vi "PixieDownloadBoot.vi"(6 "Offline analysis ?":bool, 7 "PixieBootFilePaths":T1={"Communication FPGA file for REVB (.bin file in folder \"Firmware\")"=path "C:/XIA/Pixie4/Firmware/syspixie_RevB.bin", "Communication FPGA file for REVC (.bin file in folder \"Firmware\")"=path "C:/XIA/Pixie4/Firmware/syspixie_revC.bin", "Signal proceesing FPGA file (.bin file in folder \"Firmware\")"=path "C:/XIA/Pixie4/Firmware/pixie.bin", "DSP executable code file (.bin file in folder DSP\")"=path "C:/XIA/Pixie4/DSP/PXIcode.bin", "DSP parameters file (.set file in folder \"Configuration\")"=path "C:/XIA/Pixie4/Configuration/BouncerHighNoiseDec12.txt", "DSP I/O variable file (.var file in folder \"DSP\")"=path "C:/XIA/Pixie4/DSP/PXIcode.var", "DSP memory variable file (.lst file in folder \"DSP\")"=path "C:/XIA/Pixie4/DSP/PXIcode.lst"}, 8 "error in (no error)":errorcluster, 9 "Select PXI chassis type":string(combo)="4 or 8-slot chassis", 10 "Module #":u16[](array[numeric])=[2, 3] caption="PXI Slot #" min=2 max=18 step=1, 11 "Total number of Pixie-4 modules":u16=1 min=1 max=17 step=1) -> (0 "error out":errorcluster, 3 "Return value for booting":i32)   [LabVIEW 2013, in "PixieDriver.lvlib"]
uses:
  PixieDriver.lvlib
  XIA/Pixie4/Drivers/Pixie4DLL.dll
panel:
  # "0  - boot successful\n-1  - unable to scan the PXI crate slots\n-2  - unable to read communication FPGA configuration (Rev. B)\n-3  - unable to read communication FPGA configuration (Rev. C)\n-4  - unable to read signal processing FPGA configuration\n-5  - unable to read DSP executable code\n-6  - unable to read DSP parameter values\n-7  - unable to initialize DSP parameter names\n-8  - failed to boot all modules present in the system\n-9  - failed to initialize NUMBER_MODULES\n-10- failed to initialize OFFLINE_ANALYSIS\n-11- failed to initialize MAX_NUMBER_MODULES\n-12- failed to initialize SLOT_WAVE"
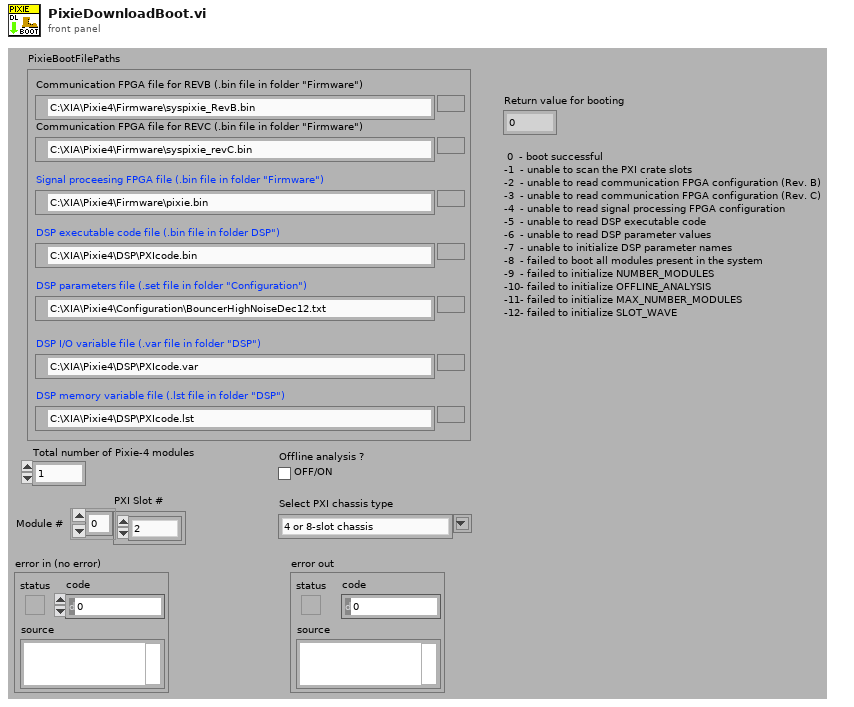
[diagram p1: front panel]
types:
  T1 = cluster{"Communication FPGA file for REVB (.bin file in folder \"Firmware\")":path, "Communication FPGA file for REVC (.bin file in folder \"Firmware\")":path, "Signal proceesing FPGA file (.bin file in folder \"Firmware\")":path, "DSP executable code file (.bin file in folder DSP\")":path, "DSP parameters file (.set file in folder \"Configuration\")":path, "DSP I/O variable file (.var file in folder \"DSP\")":path, "DSP memory variable file (.lst file in folder \"DSP\")":path}
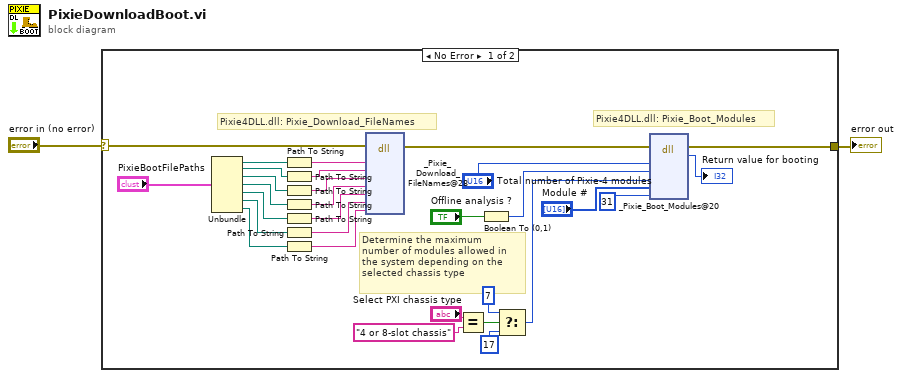
[diagram p0: block diagram]
diagram:
  n1 = case shown="No Error" "error in (no error)" {
    selector: "error in (no error)" -> [w3 w33]
    tunnel: [w4 w33] -> w2
    frame No Error {
      # "Pixie4DLL.dll: Pixie_Boot_Modules"
      # "Determine the maximum\nnumber of modules allowed in\nthe system depending on the\nselected chassis type"
      # "Pixie4DLL.dll: Pixie_Download_FileNames"
      n2 = Unbundle("PixieBootFilePaths") -> ("Communication FPGA file for REVB (.bin file in folder \"Firmware\")"=w11:path, "Communication FPGA file for REVC (.bin file in folder \"Firmware\")"=w10:path, "Signal proceesing FPGA file (.bin file in folder \"Firmware\")"=w9:path, "DSP executable code file (.bin file in folder DSP\")"=w8:path, "DSP parameters file (.set file in folder \"Configuration\")"=w7:path, "DSP I/O variable file (.var file in folder \"DSP\")"=w6:path, "DSP memory variable file (.lst file in folder \"DSP\")"=w5:path)
      n3 = Path To String(path=w11) -> (string=w26:string)
      n4 = Path To String(path=w10) -> (string=w27:string)
      n5 = Path To String(path=w9) -> (string=w28:string)
      n6 = Path To String(path=w8) -> (string=w29:string)
      n7 = Path To String(path=w7) -> (string=w30:string)
      n8 = Path To String(path=w6) -> (string=w31:string)
      n9 = Path To String(path=w5) -> (string=w32:string)
      n10 = dll-call lib="C:/XIA/Pixie4/Drivers/Pixie4DLL.dll" fn="_Pixie_Download_FileNames@28" ("Call Library Function")(error in=w3, "ComFPGAFileNameRevB"=w26, "ComFPGAFileNameRevC"=w27, "SPFPGAFileName"=w28, "DSPCodeFileName"=w29, "DSPParFileName"=w30, "DSPVarFileName"=w31, "DSPLstFileName"=w32) -> (error out=w14:errorcluster)  [unwired: 9 in, 2 out]
      n11 = Equal?(x="Select PXI chassis type", y="4 or 8-slot chassis") -> (x = y?=w18:bool)
      n12 = Boolean To (0,1)(Boolean="Offline analysis ?") -> (0, 1=w13:i16)
      n13 = Select(t=u16 7, s=w18, f=u16 17) -> (s? t:f=w15:u16)
      n14 = dll-call lib="C:/XIA/Pixie4/Drivers/Pixie4DLL.dll" fn="_Pixie_Boot_Modules@20" ("Call Library Function")(error in=w14, "TotalNumberModules"="Total number of Pixie-4 modules", "OfflineAnalysis"=w13, "MaxNumberOfModules"=w15, "PXISlotMap"="Module #", "BootPattern"=u16 31) -> (error out=w4:errorcluster, "return type"=→"Return value for booting":i32)  [unwired: 7 in, 1 out]
    }
    frame Error {
    }
  }
  "error out" <- w2
